vi "Get Target Temperature F.vi"(7 "Use Cached Data?":bool, 8 "Error In":errorcluster, 10 "Device Name":string, 11 "Nest Config":T1) -> (0 "Error Out":errorcluster, 1 "Target Temperature Low (F)":dbl, 2 "Target Temp (F)":dbl, 3 "Nest Config":T1, 5 "Target Temperature High (F)":dbl)   [LabVIEW 2013, in "LMH-Nest.lvlib"]
doc: "Get the target temperature of the specified Nest device."
uses:
  LMH-Nest.lvlib
  Private/Type Defs/Nest Config.ctl
  <vilib>/httpClient/ClientHandle.ctl
  Private/Type Defs/Session Data.ctl
  <vilib>/httpClient/LabVIEWHTTPClient.lvlib
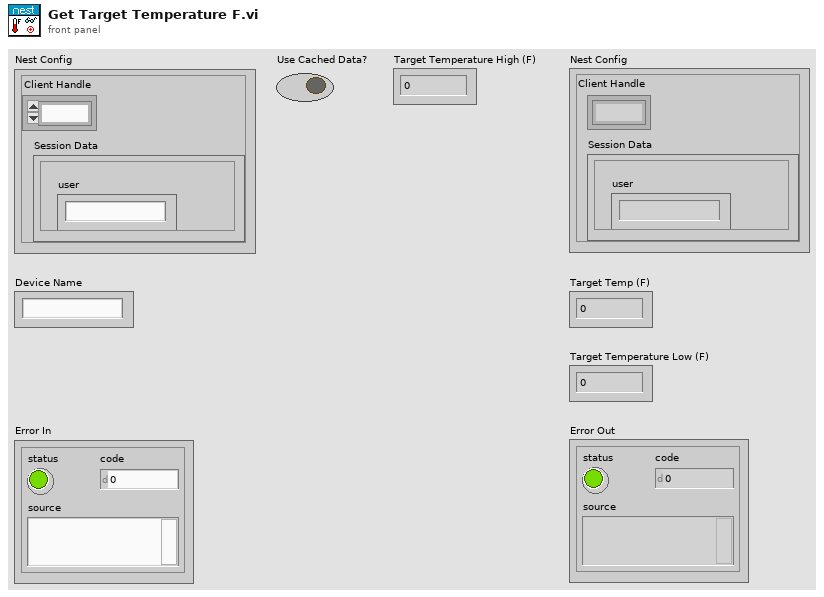
[diagram p1: front panel]
types:
  T1 = typedef "LMH-Nest.lvlib/Nest Config.ctl" = cluster{"Client Handle":T2, "Session Data":T3}
  T2 = typedef "LabVIEWHTTPClient.lvlib/ClientHandle.ctl" = refnum<k1>
  T3 = typedef "LMH-Nest.lvlib/Session Data.ctl" = cluster{"is_superuser":bool, "is_staff":bool, "urls":cluster{"transport_url":string, "rubyapi_url":string, "weather_url":string, "log_upload_url":string, "support_url":string}, "limits":cluster{"thermostats_per_structure":u32, "structures":u32, "thermostats":u32, "smoke_detectors":u32, "smoke_detectors_per_structure":u32}, "access_token":string, "userid":string, "expires_in":string, "email":string, "user":string, "language":string}
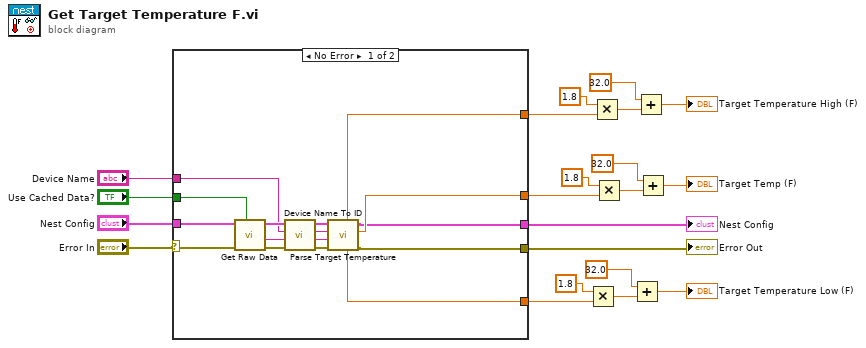
[diagram p0: block diagram]
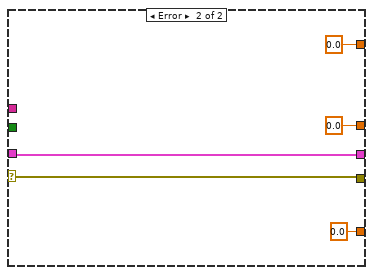
[diagram p2: hidden frame]
diagram:
  n1 = case shown="No Error" "Error In" {
    selector: "Error In" -> [w31 w42]
    tunnel: "Use Cached Data?" -> [w37 _]
    tunnel: "Nest Config" -> [w36 w41]
    tunnel: "Device Name" -> [w34 _]
    tunnel: [w26 w42] -> w18
    tunnel: [w24 w41] -> w17
    tunnel: [w25 0.0 ("Current Temp")] -> w3
    tunnel: [w23 0.0 ("Target Temperature High (C)")] -> w6
    tunnel: [w22 0.0 ("Target Temperature Low (C)")] -> w2
    frame No Error {
      n2 = call "Get Raw Data.vi"("Use Cached Data?"=w37, "Error In"=w31, "Nest Config"=w36) -> ("Error Out"=w33:errorcluster, "Data"=w32:string, "Nest Config"=w35:T1)  [unwired: 6 in]
      n3 = call "Device Name To ID.vi"("Error In"=w33, "Data"=w32, "Device Name"=w34, "Nest Config"=w35) -> ("Error Out"=w27:errorcluster, "Data"=w28:string, "Device ID"=w29:string, "Nest Config"=w30:T1)  [unwired: 4 in]
      n4 = call "Parse Target Temperature.vi"("Error In"=w27, "Data"=w28, "Device ID"=w29, "Nest Config"=w30) -> ("Error Out"=w26:errorcluster, "Target Temperature (C)"=w25:dbl, "Nest Config"=w24:T1, "Target Temperature Low (C)"=w22:dbl, "Target Temperature High (C)"=w23:dbl)  [unwired: 2 in, 1 out]
    }
    frame Error {
    }
  }
  "Error Out" <- w18
  "Nest Config" <- w17
  n5 = Multiply(x=1.8 ("y"), y=w2) -> (x*y=w11:dbl)
  n6 = Multiply(x=1.8 ("y"), y=w6) -> (x*y=w14:dbl)
  n7 = Multiply(x=1.8 ("y"), y=w3) -> (x*y=w8:dbl)
  n8 = Add(x=32.0, y=w11) -> (x+y=→"Target Temperature Low (F)":dbl)
  n9 = Add(x=32.0, y=w14) -> (x+y=→"Target Temperature High (F)":dbl)
  n10 = Add(x=32.0, y=w8) -> (x+y=→"Target Temp (F)":dbl)
